vi "Diagon Alley.vi"(8 "error in":errorcluster, 9 "Player Color":T1, 10 "Possible Moves":bool[][](array[boolean]), 11 "Board":T3[][](array[typedef])) -> (0 "error out":errorcluster, 3 "Choice Coordinates":T2)   [LabVIEW 2020]
uses:
  Reversi/Space Ring.ctl
  Reversi/Space Coordinates.ctl
  Reversi/Turn Enum.ctl
  <vilib>/numeric/Random Number (Range) I64.vi
  <vilib>/numeric/sub_Random U32.vi
  Reversi/Reversi.lvclass
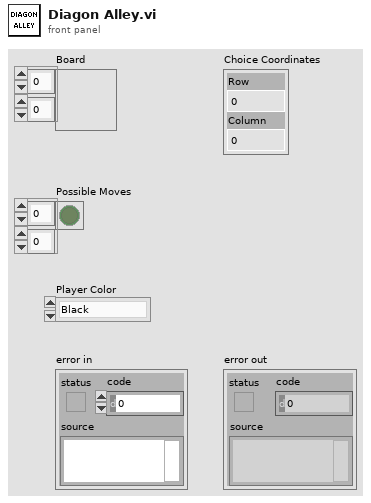
[diagram p1: front panel]
types:
  T1 = typedef "Reversi.lvlib/Reversi.lvclass/Turn Enum.ctl" = enum16{"Black", "White"}
  T2 = typedef "Reversi.lvlib/Reversi.lvclass/Space Coordinates.ctl" = cluster{"Row":i32, "Column":i32}
  T3 = typedef "Reversi.lvlib/Reversi.lvclass/Space Ring.ctl" = u16
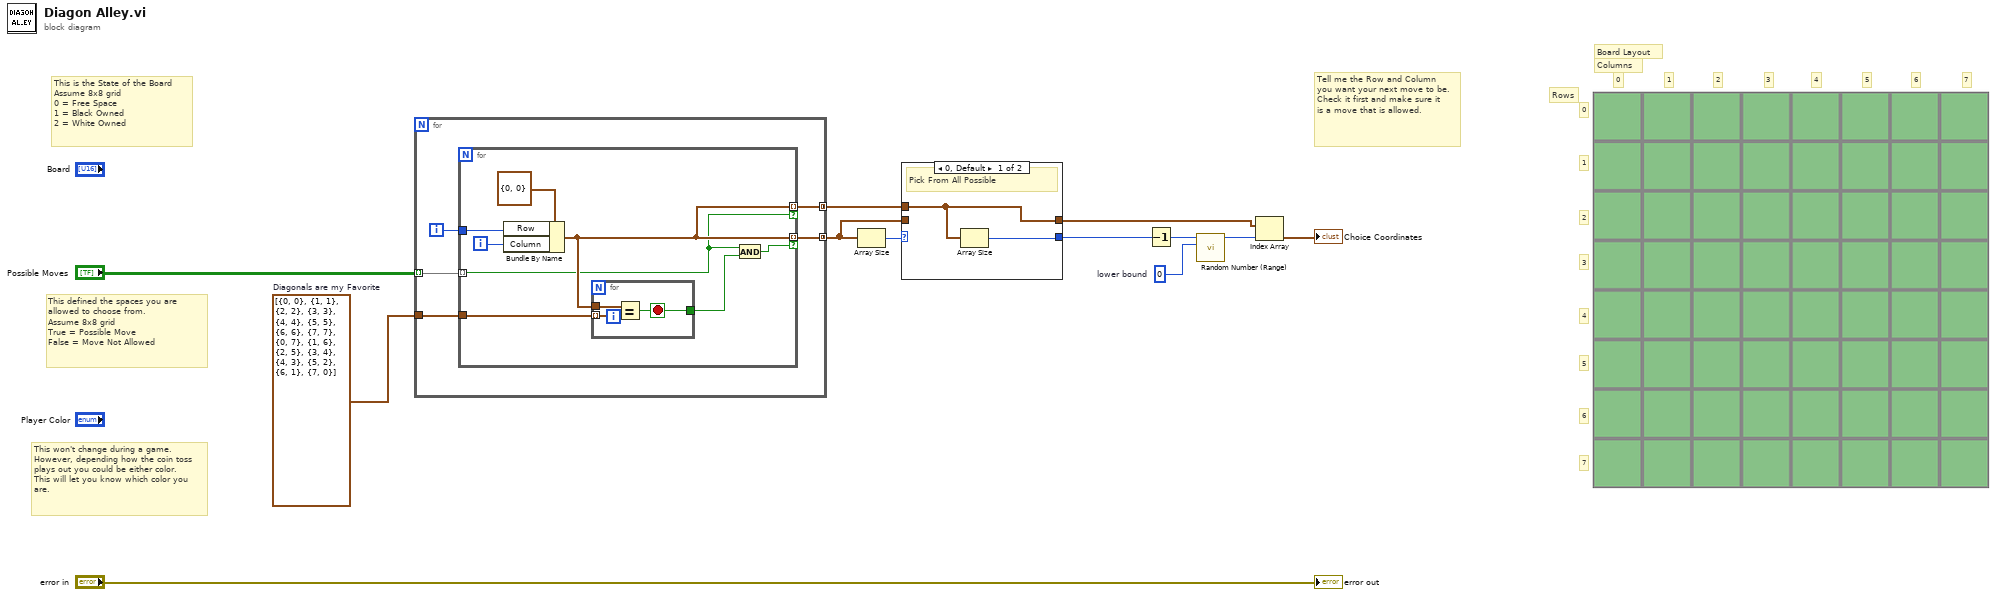
[diagram p0: block diagram]
diagram:
  w8 = i64 0  # lower bound
  w10 = T2[] [{"Row"=0, "Column"=0}, {"Row"=1, "Column"=1}, {"Row"=2, "Column"=2}, {"Row"=3, "Column"=3}, {"Row"=4, "Column"=4}, {"Row"=5, "Column"=5}, {"Row"=6, "Column"=6}, {"Row"=7, "Column"=7}, {"Row"=0, "Column"=7}, {"Row"=1, "Column"=6}, {"Row"=2, "Column"=5}, {"Row"=3, "Column"=4}, {"Row"=4, "Column"=3}, {"Row"=5, "Column"=2}, {"Row"=6, "Column"=1}, {"Row"=7, "Column"=0}]  # Diagonals are my Favorite
  # "This won't change during a game. However, depending how the coin toss plays out you could be either color. This will let you know which color you are."
  # "7"
  # "6"
  # "5"
  # "4"
  # "3"
  # "2"
  # "1"
  # "0"
  # "Rows"
  # "7"
  # "6"
  # "5"
  # "4"
  # "3"
  # "2"
  # "1"
  # "0"
  # "Columns"
  # "Board Layout"
  # "Tell me the Row and Column you want your next move to be. Check it first and make sure it is a move that is allowed."
  # "This defined the spaces you are allowed to choose from.\nAssume 8x8 grid\nTrue = Possible Move\nFalse = Move Not Allowed"
  # "This is the State of the Board\nAssume 8x8 grid\n0 = Free Space\n1 = Black Owned\n2 = White Owned"
  n1 = for {
    tunnel: "Possible Moves" -> [w17] mode=indexing
    tunnel: [w15] -> w3 mode=concatenating
    tunnel: [w14] -> w4 mode=concatenating
    tunnel: w10 -> [w13]
    i -> [w16]
    n2 = for {
      tunnel: w17 -> [w20] mode=indexing
      tunnel: w16 -> [w24]
      tunnel: [w21] -> w14 mode=indexing if=w18
      tunnel: [w21] -> w15 mode=indexing if=w20
      tunnel: w13 -> [w22]
      i -> [w23]
      n3 = Bundle By Name(cluster=T2 {"Row"=0, "Column"=0}, "Row"=w24, "Column"=w23) -> (w21:T2)
      n4 = for {
        tunnel: w22 -> [w28] mode=indexing
        tunnel: w21 -> [w27]
        tunnel: [w26] -> w19
        stop <- w26 stop-if-true
        n5 = Equal?(x=w27, y=w28) -> (x = y?=w26:bool)
      }
      n6 = And(x=w20, y=w19) -> (x .and. y?=w18:bool)
    }
  }
  n7 = Array Size(array=w4) -> (size(s)=w5:i32)
  n8 = case shown="0, Default" w5 {
    selector: w5 -> [_ w31]
    tunnel: w4 -> [_ w32]
    tunnel: w3 -> [w30 _]
    tunnel: [w30 w32] -> w2
    tunnel: [w29 w31] -> w1
    frame 0, Default {
      # "Pick From All Possible"
      n9 = Array Size(array=w30) -> (size(s)=w29:i32)
    }
    frame 1.. {
      # "Pick From Favorites"
    }
  }
  n10 = Decrement(x=w1) -> (x-1=w9:i32)
  n11 = call-poly <vilib>:"Random Number (Range).vi"("lower bound (-100)"=w8, "upper bound (100)"=w9) -> ("number"=w7:i64)  [unwired: 9 in]
  n12 = Index Array(array=w2, index=w7) -> (element=→"Choice Coordinates":T2)
  "error out" <- "error in"
